vi "Boolean.vi"() -> ()   [LabVIEW 2023]
panel:
  in  "c":bool
  out "불리언":i16
  out "불리언":bool
  in  "b":bool
  in  "a":bool
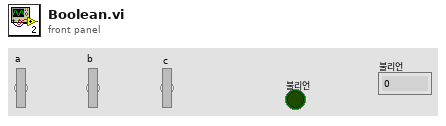
[diagram p1: front panel]
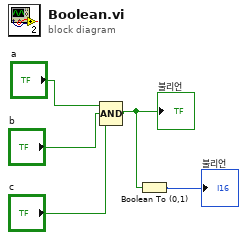
[diagram p0: block diagram]
diagram:
  n1 = Compound Arithmetic op=AND("a", "b", "c") -> (w3:bool)
  "불리언" <- w3
  n2 = Boolean To (0,1)(Boolean=w3) -> (0, 1=→"불리언":i16)
